vi "Create Notifiers.vi"(8 "error in":errorcluster) -> (0 "error out":errorcluster, 3 "Notifiers":T1)   [LabVIEW 2015, in "Notifiers.lvlib"]
doc: "Creates notifiers for handshaking and closing processes"
uses:
  Notifiers.lvlib
  Notifiers.ctl
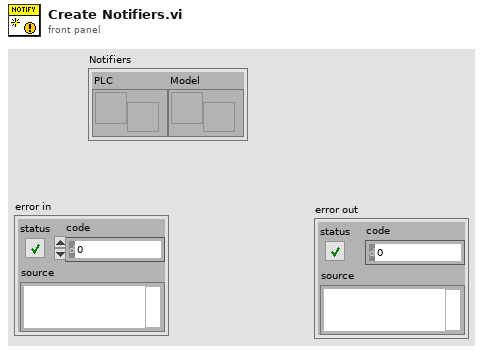
[diagram p1: front panel]
types:
  T1 = typedef "Notifiers.lvlib/Notifiers.ctl" = cluster{"PLC":refnum<notifier>, "Model":refnum<notifier>}
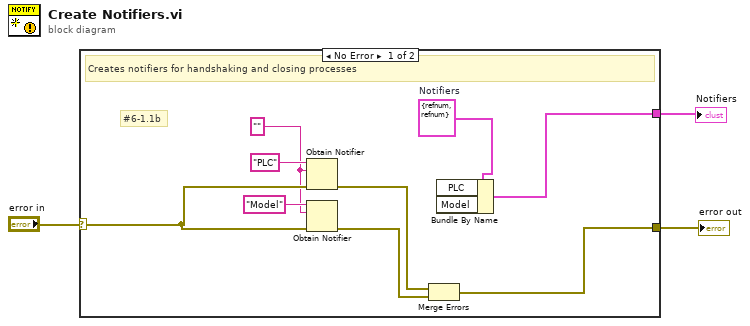
[diagram p0: block diagram]
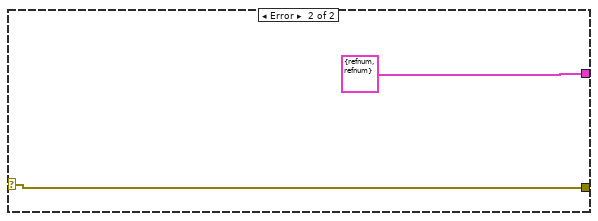
[diagram p2: hidden frame]
diagram:
  n1 = case shown="No Error" "error in" {
    selector: "error in" -> [w8 w14]
    tunnel: [w11 w14] -> w3
    tunnel: [w10 T1 {"PLC"=refnum, "Model"=refnum} ("Notifiers")] -> w2
    frame No Error {
      w4 = ""
      w7 = T1 {"PLC"=refnum, "Model"=refnum}  # Notifiers
      # "#6-1.1b"
      # "Creates notifiers for handshaking and closing processes"
      n2 = Obtain Notifier(name (unnamed)="PLC", notification data type=w4, error in (no error)=w8) -> (error out=w12:errorcluster)  [unwired: 1 in, 2 out]
      n3 = Obtain Notifier(name (unnamed)="Model", notification data type=w4, error in (no error)=w8) -> (error out=w9:errorcluster)  [unwired: 1 in, 2 out]
      n4 = Merge Errors(w12, w9) -> (w11:errorcluster)
      n5 = Bundle By Name(cluster=w7) -> (w10:T1)  [unwired: 2 in]
    }
    frame Error {
    }
  }
  "error out" <- w3
  "Notifiers" <- w2
